vi "construct_constant_array_slow.vi"(4 "Low Mass Limit":i64=256, 6 "High Mass Limit":i64=2, 7 "Low Velocity Count":i32, 8 "High Velocity Count":i32, 10 "Low Charge Limit":i16, 11 "High Charge Limit":i16) -> (3 "constants cluster":T1={"High Charge Limit"=0, "Low Charge Limit"=0, "Low Velocity Count"=0, "High Velocity Count"=0, "Low Velocity Count"=0, 26666666.59375, "High Mass Limit"=0, "Low Mass Limit"=0})   [LabVIEW 2013]
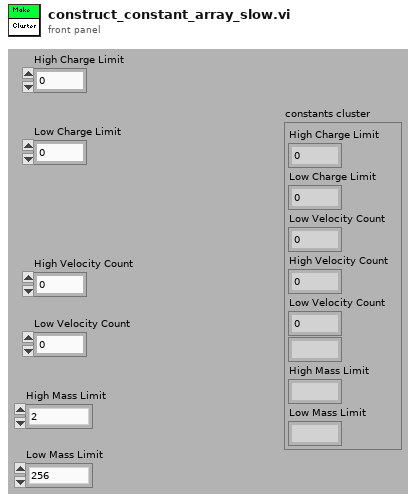
[diagram p1: front panel]
types:
  T1 = cluster{"High Charge Limit":i16, "Low Charge Limit":i16, "Low Velocity Count":i32, "High Velocity Count":i32, "Low Velocity Count":i32, fxp<+,30,25>, "High Mass Limit":i64, "Low Mass Limit":i64}
  T2 = cluster{"High Charge Limit":i16, "Low Charge Limit":i16, "Low Velocity Count":i32, "High Velocity Count":i32, "Low Velocity Count":i32, fxp<+,30,22>, "High Mass Limit":i64, "Low Mass Limit":i64}
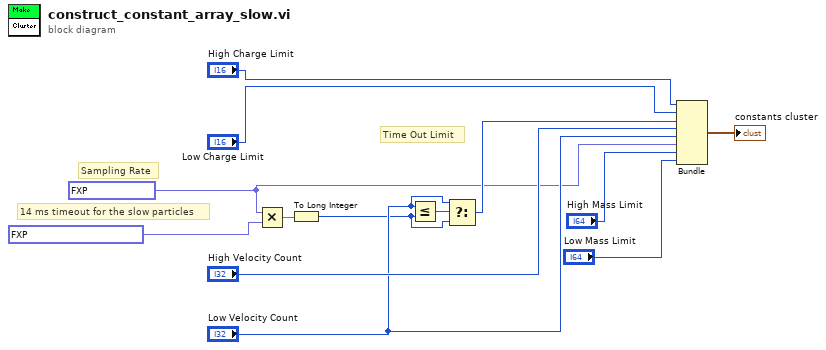
[diagram p0: block diagram]
diagram:
  w4 = fxp<+,30,22> 3333333.328125
  # "14 ms timeout for the slow particles"
  # "Sampling Rate"
  # "Time Out Limit"
  n1 = Multiply(x=w4, y=fxp<+,15,-6> 0.013959884643554688) -> (x*y=w12:fxp<+,45,16>)
  n2 = To Long Integer(number=w12) -> (32bit integer=w6:i32)
  n3 = Less Or Equal?(x="Low Velocity Count", y=w6) -> (x <= y?=w8:bool)
  n4 = Select(t="Low Velocity Count", s=w8, f=w6) -> (s? t:f=w5:i32)
  n5 = Bundle("High Charge Limit"="High Charge Limit", "Low Charge Limit"="Low Charge Limit", "Low Velocity Count"=w5, "High Velocity Count"="High Velocity Count", "Low Velocity Count"="Low Velocity Count", w4, "High Mass Limit"="High Mass Limit", "Low Mass Limit"="Low Mass Limit") -> (→"constants cluster":T2)  [unwired: 1 in]
